vi "Self-Test.vi"(8 "error in (no error)":errorcluster, 9 "Device and Axis":string, 11 "VISA resource name":refnum<visa-resource-name>) -> (0 "error out":errorcluster, 1 "Self-Test Result Message":string, 3 "VISA resource name out":refnum<visa-resource-name>)   [LabVIEW 2013, in "Zaber A Series.lvlib"]
doc: "Sends an Echo command to the device with the text \"TEST OK\". This value should be read back in the data of the response. If not, there will be an error message.\n\nThis VI requires that the Initialize VI has been called with the same serial port."
uses:
  Zaber A Series.lvlib
  Private/All Commands.ctl
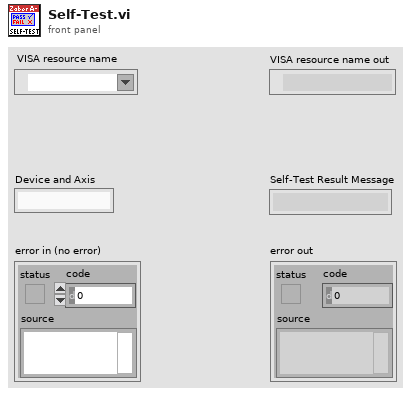
[diagram p1: front panel]
types:
  T1 = typedef "Zaber A Series.lvlib/All Commands.ctl" = string
  T2 = cluster{"Device":string, "Axis":string, "Reply Flag":string, "Status":string, "Warning Flags":string, "Data":string}[]
  T3 = cluster{"Device":string, "Axis":string, "Reply Flag":string, "Status":string, "Warning Flags":string, "Data":string}
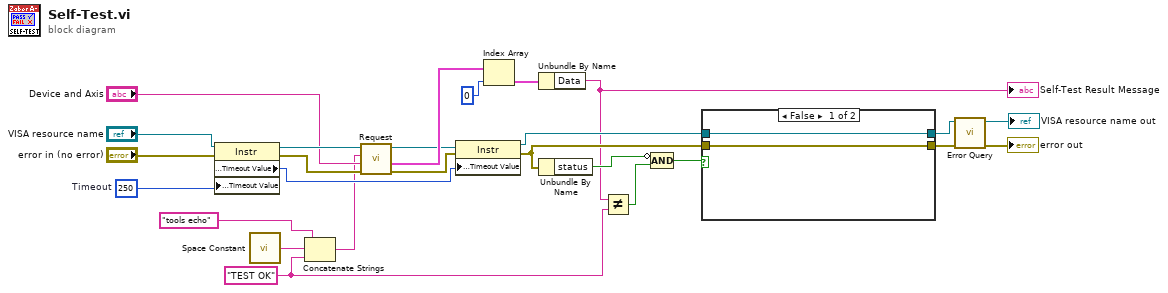
[diagram p0: block diagram]
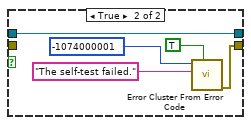
[diagram p2: hidden frame]
diagram:
  w4 = "TEST OK" ("Data")
  w22 = u32 250  # Timeout
  n1 = property class="Instr"(reference="VISA resource name", error in="error in (no error)", "General Settings:Timeout Value"=w22) -> (reference out=w14:refnum<visa-resource-name>, error out=w12:errorcluster, "General Settings:Timeout Value"=w6:u32)
  n2 = call <vilib>:"Space Constant.vi"() -> ("String"=w2:string)
  n3 = Concatenate Strings(T1 "tools echo" ("Command List"), w2, w4) -> (w1:string)
  n4 = call "Request.vi"("error in (no error)"=w12, "Device and Axis"="Device and Axis", "Command String"=w1, "VISA resource name"=w14) -> ("error out"=w13:errorcluster, "Response Bundle Array"=w9:T2, "VISA resource name out"=w5:refnum<visa-resource-name>)  [unwired: 3 in, 2 out]
  n5 = property class="Instr"(reference=w5, error in=w13, "General Settings:Timeout Value"=w6) -> (reference out=w21:refnum<visa-resource-name>, error out=w20:errorcluster)
  n6 = Index Array(array=w9, index=0) -> (element=w8:T3)
  n7 = Unbundle By Name(w8) -> ("Data"=w7:string)
  "Self-Test Result Message" <- w7
  n8 = Unbundle By Name(w20) -> ("status"=w16:bool)
  n9 = Not Equal?(x=w7, y=w4) -> (x != y?=w17:bool)
  n10 = Compound Arithmetic op=AND(invert w16, w17) -> (w15:bool)
  n11 = case shown="False" w15 {
    tunnel: w21 -> [w28 w33]
    tunnel: w20 -> [w27 _]
    tunnel: [w27 w29] -> w19
    tunnel: [w28 w33] -> w18
    frame False {
    }
    frame True {
      n12 = call <vilib>:"Error Cluster From Error Code.vi"("show call chain? (False)"=TRUE, "error message (\"\")"="The self-test failed." ("Source (VI Name)"), "error code (0)"=-1074000001 ("Code")) -> ("error out"=w29:errorcluster)  [unwired: 6 in]
    }
  }
  n13 = call "Error Query.vi"("error in (no error)"=w19, "VISA resource name"=w18) -> ("error out"=→"error out":errorcluster, "VISA resource name out"=→"VISA resource name out":refnum<visa-resource-name>)  [unwired: 6 in, 2 out]
